vi "Set RIO Resource.vi"(8 "error in":errorcluster, 10 "RIO resource in":string, 11 "FPGA addon refnum in":T1=18446744073709551615 format="%.0x") -> (0 "error out":errorcluster, 3 "FPGA addon refnum out":T1=18446744073709551615 format="%.0x")   [LabVIEW 2018, in "Scripting API.lvlib"]
uses:
  Scripting API.lvlib
  <vilib>/NI Veristand/Custom Device API/Custom Device Item Ref.ctl
  Addon/Addon Shared/Types/FG Action.ctl
  Addon/Addon Shared/SubVIs/Constants.vi
  <vilib>/NI Veristand/Custom Device API/NI VeriStand - Get Item Property.vi
  <vilib>/NI Veristand/Custom Device API/Get Item Property (Path).vi
  <vilib>/NI Veristand/Custom Device API/Get Item Property (String).vi
  <vilib>/NI Veristand/Custom Device API/Get Item Property (Boolean).vi
  <vilib>/NI Veristand/Custom Device API/NI VeriStand - Set Item Property.vi
  <vilib>/NI Veristand/Custom Device API/Set Item Property (Path).vi
  <vilib>/NI Veristand/Custom Device API/Set Item Property (String).vi
  <vilib>/NI Veristand/Custom Device API/Set Item Property (Boolean).vi
  Addon/Addon Shared/FPGA Addon Shared.lvlib
  <vilib>/NI Veristand/Custom Device API/Custom Device API.lvlib
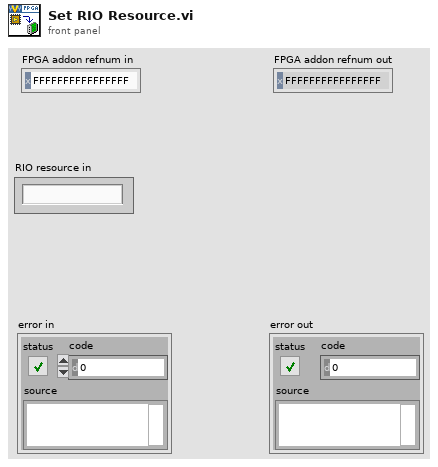
[diagram p1: front panel]
types:
  T1 = typedef "Custom Device API.lvlib/Custom Device Item Ref.ctl" = u64
  T2 = typedef "FPGA Addon Shared.lvlib/FG Action.ctl" = enum8{"GET", "SET"}
  T3 = typedef "FPGA Addon Shared.lvlib/FPGA Settings.ctl" = cluster{"Bitfile path":path, "RIO Device Address":string, "Group":bool}
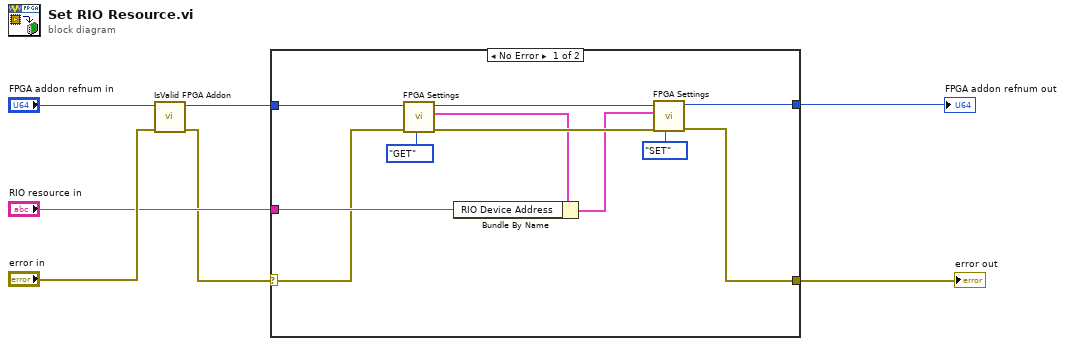
[diagram p0: block diagram]
diagram:
  n1 = call "IsValid FPGA Addon.vi"("error in"="error in", "FPGA Addon refnum in"="FPGA addon refnum in") -> ("error out"=w3:errorcluster, "FPGA Addon refnum out"=w4:T1)  [unwired: 8 in]
  n2 = case shown="No Error" w3 {
    selector: w3 -> [w10 w19]
    tunnel: "RIO resource in" -> [w14 _]
    tunnel: w4 -> [w15 w20]
    tunnel: [w9 w19] -> w2
    tunnel: [w8 w20] -> w1
    frame No Error {
      n3 = call "FPGA Settings.vi"("Action"=FG_Action."GET", "error in (no error)"=w10, "Item Ref"=w15) -> ("error out"=w17:errorcluster, "FPGA Settings"=w13:T3, "Item Ref out"=w16:T1)  [unwired: 6 in]
      n4 = Bundle By Name(cluster=w13, "RIO Device Address"=w14) -> (w12:T3)
      n5 = call "FPGA Settings.vi"("Action"=FG_Action."SET", "error in (no error)"=w17, "FPGA Settings"=w12, "Item Ref"=w16) -> ("error out"=w9:errorcluster, "Item Ref out"=w8:T1)  [unwired: 5 in, 1 out]
    }
    frame Error {
    }
  }
  "error out" <- w2
  "FPGA addon refnum out" <- w1
